vi "AddNode.vi"(8 "error in (no error)":errorcluster caption="错误输入（无错误）", 9 "Index":i32, 10 "Node*":refnum<data-value>, 11 "PanelRootNode 输入":refnum<class "PanelRootNode.lvclass"> caption="DNL_LabVIEW Object in") -> (0 "error out":errorcluster caption="错误输出", 3 "PanelRootNode 输出":refnum<class "PanelRootNode.lvclass"> caption="DNL_LabVIEW Object out")   [LabVIEW 2013, in "PanelRootNode.lvclass"]
uses:
  PanelRootNode.lvclass
  PanelObject/PanelObject.lvclass
  PanelRootNode.lvclass/PanelRootNode.ctl
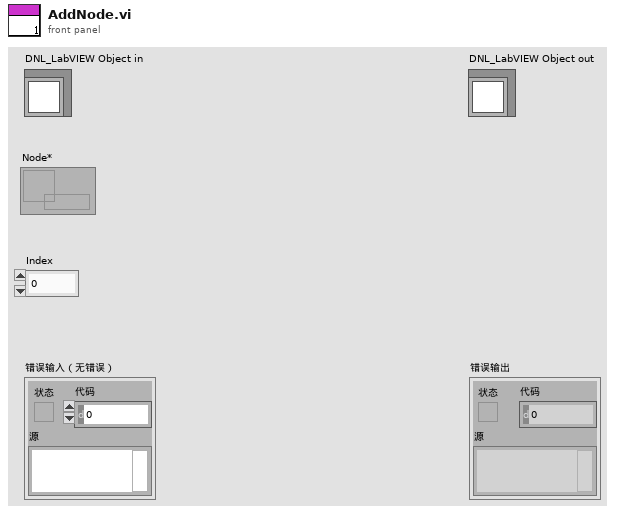
[diagram p1: front panel]
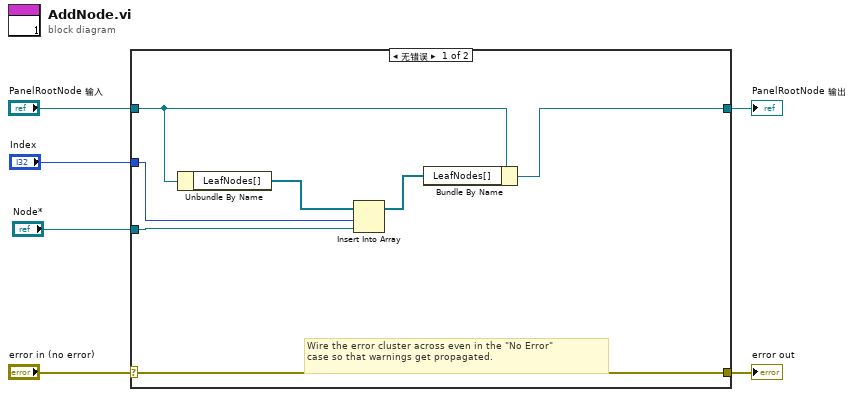
[diagram p0: block diagram]
diagram:
  n1 = case shown="无错误" "error in (no error)" {
    selector: "error in (no error)" -> [w13 w15]
    tunnel: [w13 w15] -> w5
    tunnel: [w7 w14] -> w3
    tunnel: "PanelRootNode 输入" -> [w8 w14]
    tunnel: "Node*" -> [w10 _]
    tunnel: "Index" -> [w11 _]
    frame No Error {
      # "Wire the error cluster across even in the \"No Error\"\ncase so that warnings get propagated."
      n2 = Unbundle By Name(w8) -> ("LeafNodes[]"=w12:refnum<data-value>[])
      n3 = Insert Into Array(array=w12, index=w11, new element=w10) -> (w9:refnum<data-value>[])
      n4 = Bundle By Name(cluster=w8, "LeafNodes[]"=w9) -> (w7:refnum<class "PanelRootNode.lvclass">)
    }
    frame Error {
    }
  }
  "error out" <- w5
  "PanelRootNode 输出" <- w3
